vi "AppConfigXMLToType.vi"(8 "error in (no error)":errorcluster, 10 "Config in":variant, 11 "RingdownPlugin in":refnum<class "RingdownPlugin.lvclass">) -> (0 "error out":errorcluster, 3 "RingdownPlugin out":refnum<class "RingdownPlugin.lvclass">)   [LabVIEW 2014, in "AppPlugins.lvlib" / "RingdownPlugin.lvclass"]
uses:
  RingdownPlugin.lvclass
  PublicAPI/TypeDef/RingdownConfig.ctl
  RingdownPlugin.lvclass/RingdownPlugin.ctl
  Accessors/Write RingdownConfig.vi
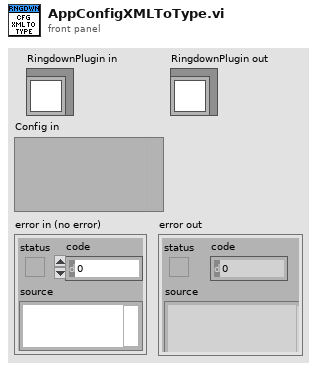
[diagram p1: front panel]
types:
  T1 = typedef "AppPlugins.lvlib/RingdownPlugin.lvclass/RingdownConfig.ctl" = cluster{"Config":cluster{"Addmod":i32, "Scalmod":i32, "Lpocon":i32, "Pircon":i32, "Dmodes":i32, "Lpmcon":u16, "Lpacon":u16, "Fbcon":u16, "Ordcon":i32, "Trimre":dbl, "Ftrimh":dbl, "Ftriml":dbl}, "Window":cluster{"StOffset":i32, "EndOffset":i32, "Length":i32}, "V index":i32, "I index":i32, "PosSeq":bool}
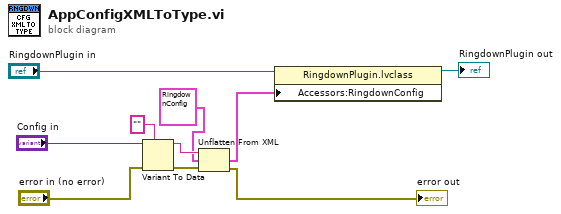
[diagram p0: block diagram]
diagram:
  n1 = Variant To Data(error in="error in (no error)", type="", Variant="Config in") -> (data=w7:string, error out=w6:errorcluster)
  n2 = Unflatten From XML(xml string=w7, type=T1 {"Config"={"Addmod"=-1, "Scalmod"=0, "Lpocon"=-1, "Pircon"=-1, "Dmodes"=0, "Lpmcon"=3, "Lpacon"=1, "Fbcon"=1, "Ordcon"=1, "Trimre"=-1.0, "Ftrimh"=-1.0, "Ftriml"=-1.0}, "Window"={"StOffset"=0, "EndOffset"=1000, "Length"=1000}, "V index"=0, "I index"=3, "PosSeq"=FALSE} ("RingdownConfig"), error in (no error)=w6) -> (value=w1:T1, error out=→"error out":errorcluster)
  n3 = property class="RingdownPlugin.lvclass"(reference="RingdownPlugin in", "Accessors:RingdownConfig"=w1) -> (reference out=→"RingdownPlugin out":refnum<class "RingdownPlugin.lvclass">)  [unwired: 1 in, 1 out]
